vi "Write Spreadsheet String.vi"(7 "prompt":string, 8 "error in":errorcluster, 9 "append to file? (new file:F)":bool, 10 "spreadsheet string":string, 11 "file path (dialog if empty)":path) -> (0 "error out":errorcluster, 3 "path":path)   [LabVIEW 2020]
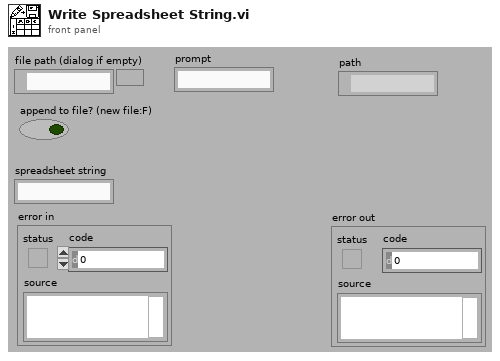
[diagram p1: front panel]
types:
  T1 = enum16{"open", "replace", "create", "open or create", "replace or create", "replace or create with confirmation"}
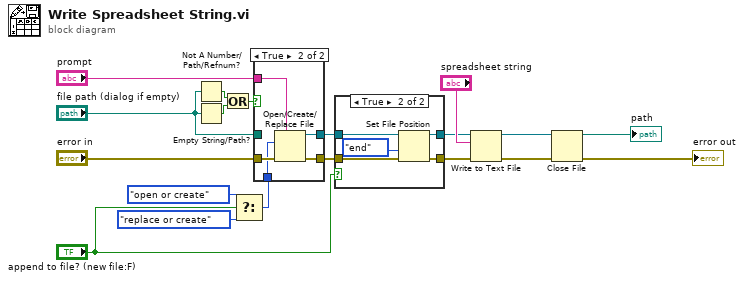
[diagram p0: block diagram]
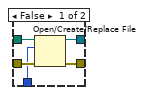
[diagram p3: hidden frame]
diagram:
  n1 = Not A Number/Path/Refnum?(number/path/refnum="file path (dialog if empty)") -> (NaN/Path/Refnum?=w11:bool)
  n2 = Empty String/Path?(string/path="file path (dialog if empty)") -> (empty?=w12:bool)
  n3 = Or(x=w11, y=w12) -> (x .or. y?=w10:bool)
  n4 = Select ("function")(t=T1."open or create" ("operation (0:open)"), s="append to file? (new file:F)", f=T1."replace or create" ("operation (0:open)")) -> (s? t:f=w6:T1)
  n5 = case shown="True" w10 {
    tunnel: "prompt" -> [_ w27]
    tunnel: "error in" -> [w24 w28]
    tunnel: [w23 w29] -> w4
    tunnel: [w22 w26] -> w3
    tunnel: "file path (dialog if empty)" -> [w21 _]
    tunnel: w6 -> [w20 w25]
    frame False {
      n6 = Open/Create/Replace File(file path (use dialog)=w21, error in=w24, operation (0:open)=w20) -> (refnum out=w22:refnum<file>, error out=w23:errorcluster)  [unwired: 3 in, 1 out]
    }
    frame True {
      n7 = Open/Create/Replace File(error in=w28, prompt=w27, operation (0:open)=w25) -> (refnum out=w26:refnum<file>, error out=w29:errorcluster)  [unwired: 3 in, 1 out]
    }
  }
  n8 = case shown="True" "append to file? (new file:F)" {
    tunnel: w4 -> [w30 w36]
    tunnel: [w30 w35] -> w5
    tunnel: w3 -> [w31 w33]
    tunnel: [w31 w34] -> w2
    frame False {
    }
    frame True {
      n9 = Set File Position(refnum=w33, from (0:start)=enum16{"start", "end", "current"}."end", error in=w36) -> (refnum out=w34:refnum<file>, error out=w35:errorcluster)  [unwired: 1 in]
    }
  }
  n10 = Write to Text File(file (use dialog)=w2, text="spreadsheet string", error in=w5) -> (refnum out=w15:refnum<file>, error out=w13:errorcluster)  [unwired: 1 in, 1 out]
  n11 = Close File(refnum=w15, error in=w13) -> (path=→"path":path, error out=→"error out":errorcluster)
